vi "NicmosStop.vi"(9 "error in (no error)":errorcluster caption="error out (no error)") -> (6 "error out":errorcluster)   [LabVIEW 2009]
uses:
  Controls/NICMOS.COMMAND.ctl
  Controls/NICMOS.COMMANDBASIC.ctl
  Controls/NICMOS.READOUT.ctl
  Controls/NICMOS.FILTERCOMMAND.ctl
  Controls/NICMOS.FILTER.ctl
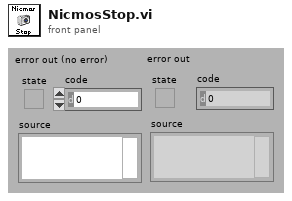
[diagram p1: front panel]
types:
  T1 = typedef "NICMOS.COMMAND.ctl" = cluster{"Command":T2, "READOUT":T3, "FILTERCOMMAND":T4, "ACQUISITION":i32, "Done":refnum<k4>}
  T2 = typedef "NICMOS.COMMANDBASIC.ctl" = enum16{"WRITE BANKS", "SET FILTER", "HOME FILTER", "QUERY TEMP", "CONFIGURE", "START", "ACQUISITION", "STOP", "QUIT"}
  T3 = typedef "NICMOS.READOUT.ctl" = cluster{"Readout":i32, "Deglitch":i32, "Framerate":dbl[unit], "Bank":i32}
  T4 = typedef "NICMOS.FILTERCOMMAND.ctl" = cluster{"FILTER":T5, "INIT":bool}
  T5 = typedef "NICMOS.FILTER.ctl" = string
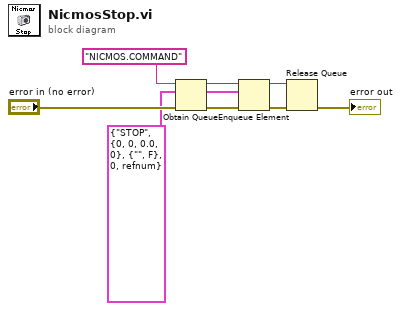
[diagram p0: block diagram]
diagram:
  w1 = T1 {"Command"=enum."STOP", "READOUT"={"Readout"=0, "Deglitch"=0, "Framerate"=0.0, "Bank"=0}, "FILTERCOMMAND"={"FILTER"="", "INIT"=FALSE}, "ACQUISITION"=0, "Done"=refnum} ("NicmosCommand")
  n1 = Obtain Queue(name (unnamed)="NICMOS.COMMAND" ("nom (aucun)"), element data type=w1, error in (no error)="error in (no error)") -> (queue out=w3:refnum<queue>, error out=w7:errorcluster)  [unwired: 2 in, 1 out]
  n2 = Enqueue Element(queue=w3, element=w1, error in (no error)=w7) -> (queue out=w2:refnum<queue>, error out=w6:errorcluster)  [unwired: 1 in, 1 out]
  n3 = Release Queue(queue=w2, error in (no error)=w6) -> (error out=→"error out":errorcluster)  [unwired: 1 in, 2 out]
